vi "ReadNearFar.vi"(1 "本次文件名":string) -> ()   [LabVIEW 2018]
uses:
  Init/AllPath.vi
  <vilib>/Utility/file.llb/Read Delimited Spreadsheet (string).vi
  HistoryFile.vi
panel:
  out "发散角Y":string
  out "发散角X":string
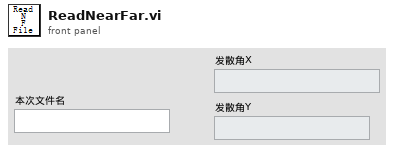
[diagram p1: front panel]
types:
  T1 = typedef "Image Type" = u32
  T2 = cluster{"能量/功率":path, " 示波器":path, " 光谱仪":path, "偏振":path, "近远场":cluster{" 近场图片":path, " 远场图片":path, "发散角数据":path}, "参数":path, " 基路径":path, "文件名信息":path, "输出模板路径":path, "输出报告路径":path}
  T3 = typedef "IMAQ Image.ctl" = refnum<image>
  T4 = cluster{"近场图":T3, " 远场图":T3, "发散角X":string, "发散角Y":string}
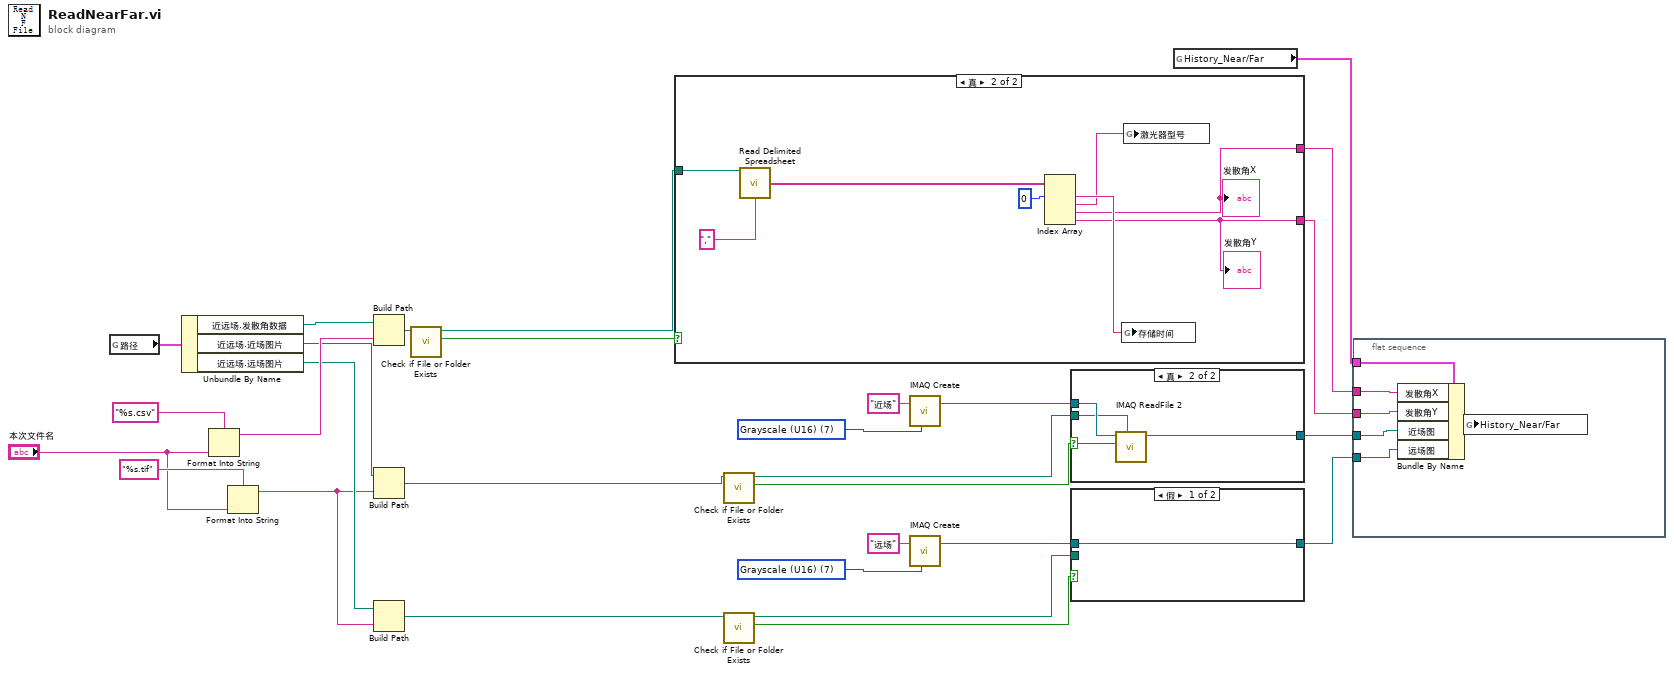
[diagram p0: block diagram]
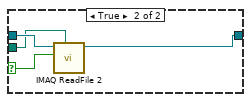
[diagram p2: hidden frame]
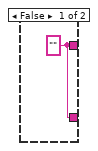
[diagram p4: hidden frame]
diagram:
  w10 = T1 7 items=["Grayscale (U8)", "Grayscale (I16)", "Grayscale (SGL)", "Complex (CSG)", "RGB (U32)", "HSL (U32)", "RGB (U64)", "Grayscale (U16)"] ("Image Type")
  w15 = T1 7 items=["Grayscale (U8)", "Grayscale (I16)", "Grayscale (SGL)", "Complex (CSG)", "RGB (U32)", "HSL (U32)", "RGB (U64)", "Grayscale (U16)"] ("Image Type")
  n1 = global read "AllPath.vi" "路径"() -> (w29:T2)
  n2 = Unbundle By Name(w29) -> ("近远场.发散角数据"=w28:path, "近远场.近场图片"=w20:path, "近远场.远场图片"=w8:path)
  n3 = Format Into String(format string="%s.csv" ("格式字符串"), "本次文件名") -> (resulting string=w26:string)  [unwired: 2 in, 1 out]
  n4 = Format Into String(format string="%s.tif" ("格式字符串"), "本次文件名") -> (resulting string=w7:string)  [unwired: 2 in, 1 out]
  n5 = Build Path(base path=w28, name or relative path=w26) -> (appended path=w25:path)
  n6 = Build Path(base path=w20, name or relative path=w7) -> (appended path=w19:path)
  n7 = Build Path(base path=w8, name or relative path=w7) -> (appended path=w6:path)
  n8 = call <vilib>:"Check if File or Folder Exists.vi"("path"=w25) -> ("file or folder exists?"=w23:bool, "dup path"=w24:path)  [unwired: 8 in, 1 out]
  n9 = case shown="真" w23 {
    tunnel: w24 -> [_ w33]
    tunnel: [w30 w32] -> w12
    tunnel: [w30 w31] -> w13
    frame False {
      w30 = ""
    }
    frame True {
      n10 = call-poly <vilib>:"Read Delimited Spreadsheet.vi"("file path (dialog if empty)"=w33, "delimiter (\\t)"="," ("delimiter (\\t)")) -> ("first row"=w38:string[])  [unwired: 8 in, 5 out]
      n11 = Index Array(array=w38, index #1=0 ("索引")) -> (element #1=w35:string, element #2=w34:string, element #3=w31:string, element #4=w32:string)  [unwired: 3 in]
      "发散角X" <- w31
      "发散角Y" <- w32
      n12 = global write "HistoryFile.vi" "存储时间"(w35) -> ()
      n13 = global write "HistoryFile.vi" "激光器型号"(w34) -> ()
    }
  }
  n14 = call <vilib>:"Check if File or Folder Exists.vi"("path"=w19) -> ("file or folder exists?"=w18:bool, "dup path"=w16:path)  [unwired: 8 in, 1 out]
  n15 = call <vilib>:"Check if File or Folder Exists.vi"("path"=w6) -> ("file or folder exists?"=w5:bool, "dup path"=w4:path)  [unwired: 8 in, 1 out]
  n16 = call "IMAQ Create"("Image Name"="近场", "Image Type"=w15) -> ("New Image"=w1:T3)  [unwired: 3 in, 1 out]
  n17 = call "IMAQ Create"("Image Name"="远场", "Image Type"=w10) -> ("New Image"=w9:T3)  [unwired: 3 in, 1 out]
  n18 = case shown="真" w18 {
    selector: w18 -> [_ w43]
    tunnel: w1 -> [w39 w42]
    tunnel: [w39 w40] -> w2
    tunnel: w16 -> [_ w41]
    frame False {
    }
    frame True {
      n19 = call "IMAQ ReadFile 2"("File Path"=w41, "Load Color Palette? (No)"=w43, "Image"=w42) -> ("Image Out"=w40:T3)  [unwired: 4 in, 4 out]
    }
  }
  n20 = case shown="假" w5 {
    selector: w5 -> [_ w48]
    tunnel: w9 -> [w44 w47]
    tunnel: [w44 w46] -> w3
    tunnel: w4 -> [_ w45]
    frame False {
    }
    frame True {
      n21 = call "IMAQ ReadFile 2"("File Path"=w45, "Load Color Palette? (No)"=w48, "Image"=w47) -> ("Image Out"=w46:T3)  [unwired: 4 in, 4 out]
    }
  }
  n22 = global read "HistoryFile.vi" "History_Near/Far"() -> (w14:T4)
  n23 = flat-sequence {
    tunnel: w14 -> [w54]
    tunnel: w13 -> [w53]
    tunnel: w12 -> [w52]
    tunnel: w2 -> [w49]
    tunnel: w3 -> [w50]
    frame #0 {
      n24 = Bundle By Name(cluster=w54, "发散角X"=w53, "发散角Y"=w52, "近场图"=w49, "远场图"=w50) -> (w51:T4)
      n25 = global write "HistoryFile.vi" "History_Near/Far"(w51) -> ()
    }
  }
